vi "test_Adding Static Scalar Input Channels.vi"(8 "error in (no error)":errorcluster, 11 "TestCase in":refnum<class "FPGA Addon Adding a Channel Item.lvclass">) -> (0 "error out":errorcluster, 3 "TestCase out":refnum<class "FPGA Addon Adding a Channel Item.lvclass">)   [LabVIEW 2019, in "FPGA Addon Adding a Channel Item.lvclass"]
uses:
  FPGA Addon Adding a Channel Item.lvclass
  <vilib>/NI VeriStand/Custom Device API/Custom Device Channel.ctl
  <vilib>/NI VeriStand/Custom Device API/Custom Device Channel Type.ctl
  Addon/Addon Shared/Types/FG Action.ctl
  Addon/Addon System Explorer/Types/Channel Type.ctl
  FPGA Addon Adding a Channel Item.lvclass/FPGA Addon Adding a Channel Item.ctl
  Addon/Addon Shared/SubVIs/Constants.vi
  <vilib>/NI VeriStand/Custom Device Tools/Custom Device Utility Library/NI VeriStand - Search for Item by GUID.vi
  <vilib>/NI/NI VeriStand Advanced SysDef API/SysDef API/SysDef.Property.Get.vi
  <vilib>/NI/NI VeriStand Advanced SysDef API/_SubVIs/SysDef.Property.Get.Variant.vi
  <vilib>/NI/NI VeriStand Advanced SysDef API/SysDef API/SysDef.Property.Set.vi
  <vilib>/NI/NI VeriStand Advanced SysDef API/_SubVIs/SysDef.Property.Set.Variant.vi
  <vilib>/NI/NI VeriStand Advanced SysDef API/_SubVIs/SysDef.Search.GUIDs.vi
  <vilib>/addons/_JKI Toolkits/VI Tester/TestCase.llb/TestCase.lvclass
  Addon/Addon System Explorer/FPGA Addon System Explorer.lvlib
  Addon/Addon Shared/FPGA Addon Shared.lvlib
  <vilib>/NI VeriStand/Custom Device Tools/Custom Device Utility Library/Custom Device Utility Library.lvlib
  <vilib>/NI/NI VeriStand Advanced SysDef API/SysDef API/Advanced System Definition.lvlib
  <vilib>/NI VeriStand/Custom Device API/Custom Device API.lvlib
  C:/Program Files (x86)/National Instruments/LabVIEW 2019/vi.lib/addons/_JKI Toolkits/VI Tester/TestCase.llb/TestCase.lvclass
panel:
  out "GUIDs":string[](array[string])
  out "Channels":T1[](array[typedef])
  in  "remove":bool
  in  "add":bool
  out "Names":string[](array[string])
  in  "Available Registers":i32[](listbox)
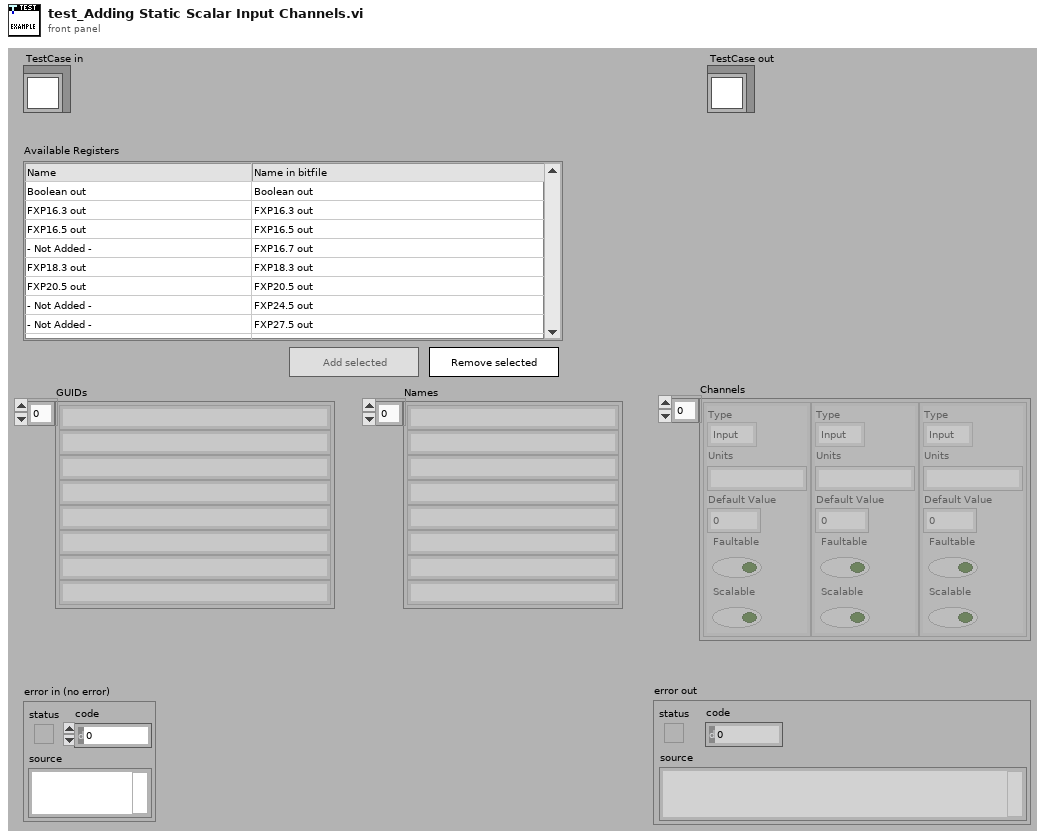
[diagram p1: front panel]
types:
  T1 = typedef "Custom Device API.lvlib/Custom Device Channel.ctl" = cluster{"Type":T2, "Units":string, "Default Value":dbl, "Faultable":bool, "Scalable":bool}
  T2 = typedef "Custom Device API.lvlib/Custom Device Channel Type.ctl" = enum16{"Input", "Output"}
  T3 = typedef "FPGA Addon System Explorer.lvlib/Channel Type.ctl" = enum16{"Write Channel", "Read Channel", "Write Waveform", "Read Waveform"}
  T4 = typedef "FPGA Addon Shared.lvlib/FG Action.ctl" = enum8{"GET", "SET"}
  T5 = typedef "Custom Device API.lvlib/Custom Device Item Ref.ctl" = u64
  T6 = typedef "FPGA Addon Shared.lvlib/Register Information.ctl" = cluster{"Name":string, "Data Type":T7, "Default Value":variant}
  T7 = typedef "FPGA Addon Shared.lvlib/Data Type.ctl" = enum8{"<Null>", "I8", "I16", "I32", "I64", "U8", "U16", "U32", "U64", "SGL", "Boolean", "Analog PWM In Settings", "Analog PWM In", "Digital PWM In Settings", "Digital PWM In", "Digital PWM Out", "Sine Out", "FXP+/-24.5", "FXP+/-16.5", "FXP+/-32.8", "FXP+/-64.32", "FXP+/-16.7", "FXP+/-20.5", "FXP+/-27.5", "FXP+/-32.16", "FXP+16.3", "FXP+18.3", "Digital Static In", "Digital Static Out", "Digital Static In Settings", "Digital WSS Out", "Quad Encoder Settings", "Quad Encoder In", "Group"}
  T8 = typedef "FPGA Addon System Explorer.lvlib/Listbox Cluster.ctl" = cluster{"add":refnum<vi>, "remove":refnum<vi>, "Listbox":refnum<vi>, "selected":i32[], "not present":i32[], "listbox text":string[][], "Section Ref":T5}
  T9 = typedef "Advanced System Definition.lvlib/TreeItem.Info.ctl" = cluster{"Name":string, "Description":string, "GUID":string, "Is Channel":bool, "Channel":T1, "Is Waveform":bool, "Waveform":T10}
  T10 = typedef "Custom Device API.lvlib/Custom Device Waveform.ctl" = cluster{"Data Type":T11, "Units":string}
  T11 = typedef "Custom Device API.lvlib/Custom Device Waveform DataType.ctl" = enum16{"Double", "Complex Double"}
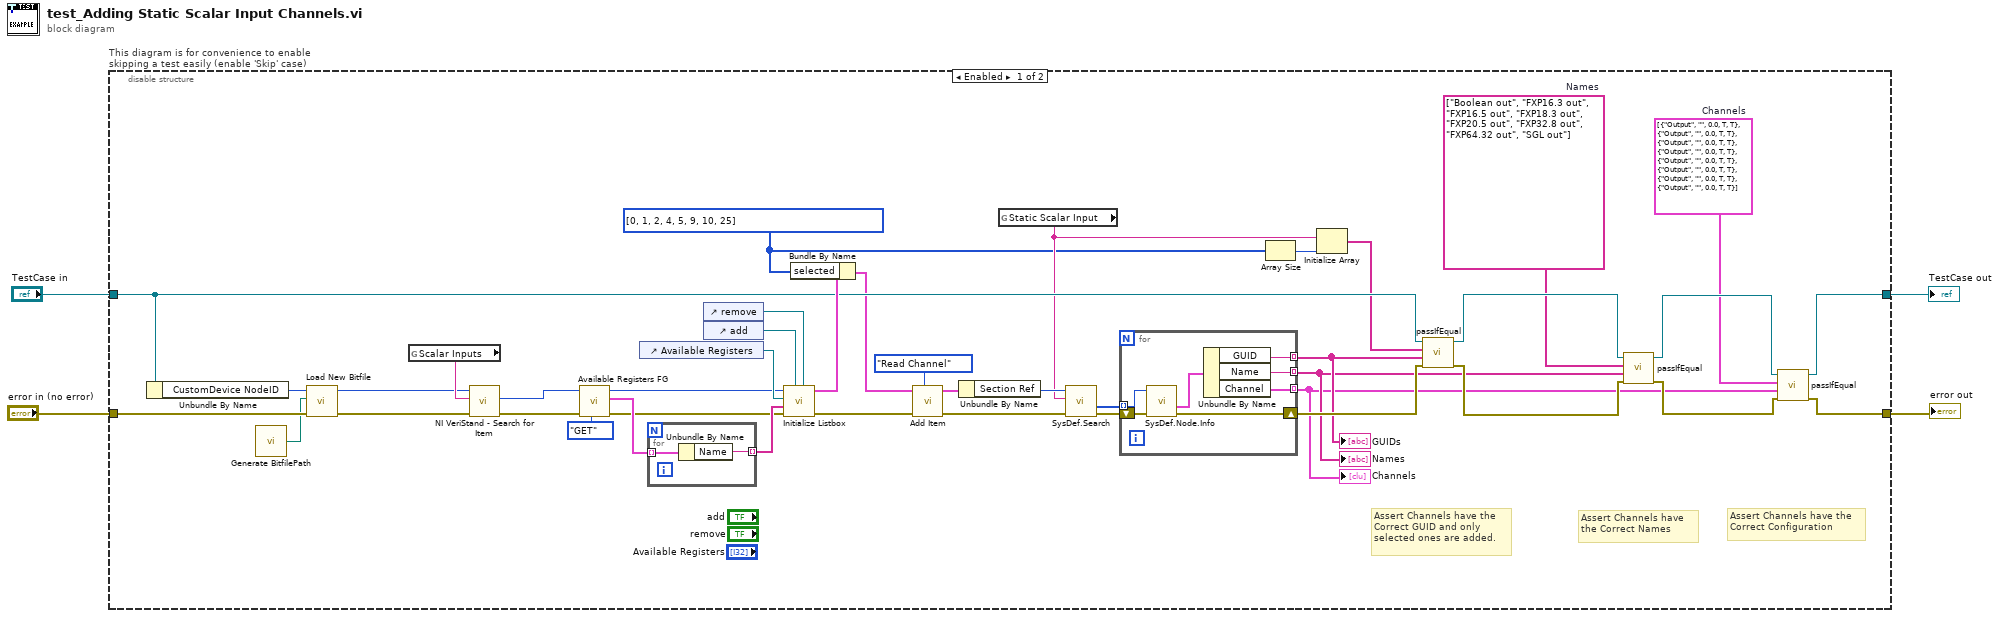
[diagram p0: block diagram]
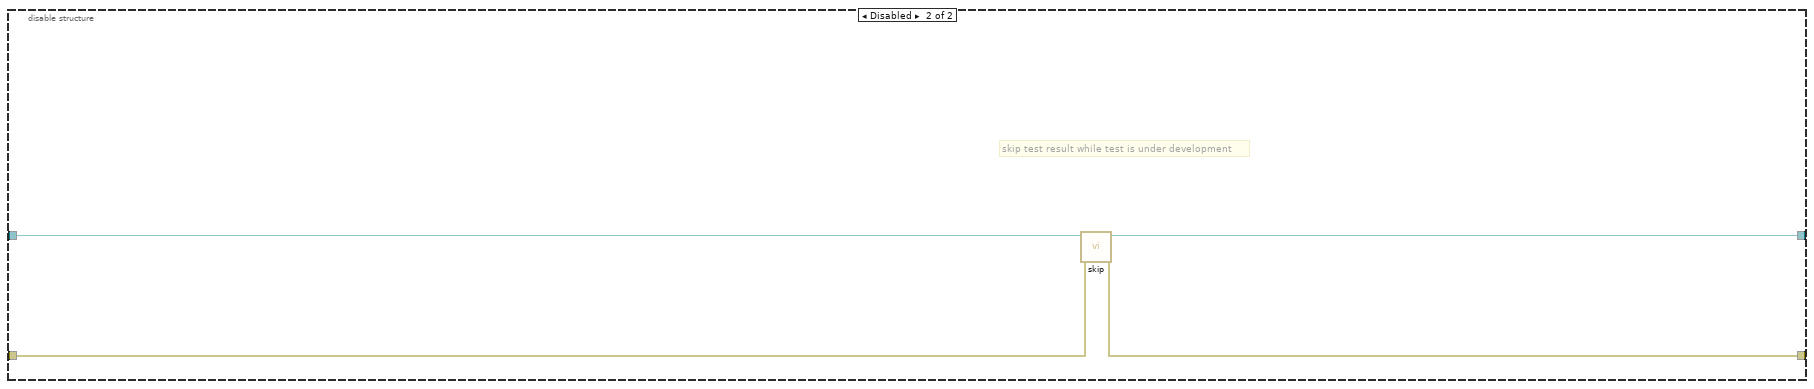
[diagram p2: hidden frame]
diagram:
  n1 = disable-structure "This diagram is for convenience to enable skipping a test easily (enable 'Skip' case)" shown="Enabled" {
    disable-tunnel: "TestCase in" -> [w26 w59]
    disable-tunnel: [w22 w57] -> w1
    disable-tunnel: [w19 w58] -> w3
    disable-tunnel: "error in (no error)" -> [w15 w56]
    frame Enabled {
      w17 = T1[] [{"Type"=enum."Output", "Units"="", "Default Value"=0.0, "Faultable"=TRUE, "Scalable"=TRUE}, {"Type"=enum."Output", "Units"="", "Default Value"=0.0, "Faultable"=TRUE, "Scalable"=TRUE}, {"Type"=enum."Output", "Units"="", "Default Value"=0.0, "Faultable"=TRUE, "Scalable"=TRUE}, {"Type"=enum."Output", "Units"="", "Default Value"=0.0, "Faultable"=TRUE, "Scalable"=TRUE}, {"Type"=enum."Output", "Units"="", "Default Value"=0.0, "Faultable"=TRUE, "Scalable"=TRUE}, {"Type"=enum."Output", "Units"="", "Default Value"=0.0, "Faultable"=TRUE, "Scalable"=TRUE}, {"Type"=enum."Output", "Units"="", "Default Value"=0.0, "Faultable"=TRUE, "Scalable"=TRUE}, {"Type"=enum."Output", "Units"="", "Default Value"=0.0, "Faultable"=TRUE, "Scalable"=TRUE}]  # Channels
      w23 = string[] ["Boolean out", "FXP16.3 out", "FXP16.5 out", "FXP18.3 out", "FXP20.5 out", "FXP32.8 out", "FXP64.32 out", "SGL out"]  # Names
      w6 = i32[] [0, 1, 2, 4, 5, 9, 10, 25] ("selected")
      # "Assert Channels have the Correct Configuration"
      # "Assert Channels have the Correct Names"
      # "Assert Channels have the Correct GUID and only selected ones are added."
      n2 = Unbundle By Name(w26) -> ("CustomDevice NodeID"=w14:u64)
      n3 = call "Generate BitfilePath.vi"() -> ("Bitfile path"=w13:path)
      n4 = call "Load New Bitfile.vi"("error in (no error)"=w15, "NewVal"=w13, "Item Ref in"=w14) -> ("error out"=w16:errorcluster, "Section Ref out"=w12:T5)  [unwired: 7 in]
      n5 = global read "Constants.vi" "Scalar Inputs"() -> (w40:string)
      n6 = call-poly <vilib>:"NI VeriStand - Search for Item.vi"("error in"=w16, "Item GUID"=w40, "Section Ref in"=w12) -> ("error out"=w39:errorcluster, "Item Ref"=w34:T5)  [unwired: 5 in, 2 out]
      n7 = call "Available Registers FG.vi"("Action"=FG_Action."GET", "error in (no error)"=w39, "Item Ref"=w34) -> ("error out"=w38:errorcluster, "Available Registers"=w44:T6[], "Item Ref out"=w36:T5)  [unwired: 6 in]
      n8 = control-ref of="Available Registers"() -> (w46:refnum<vi>)
      n9 = for {
        tunnel: w44 -> [w48] mode=indexing
        tunnel: [w47] -> w43 mode=indexing
        n10 = Unbundle By Name(w48) -> ("Name"=w47:string)
      }
      n11 = control-ref of="remove"() -> (w31:refnum<vi>)
      n12 = control-ref of="add"() -> (w32:refnum<vi>)
      n13 = call "Initialize Listbox.vi"("remove"=w31, "add"=w32, "error in (no error)"=w38, "Names"=w43, "Listbox"=w46, "Item Ref"=w36) -> ("error out"=w37:errorcluster, "Listbox Refs"=w41:T8)  [unwired: 4 in]
      n14 = Bundle By Name(cluster=w41, "selected"=w6) -> (w10:T8)
      n15 = call "Add Item.vi"("Action"=Channel_Type."Read Channel", "error in (no error)"=w37, "Listbox Refs in"=w10) -> ("error out"=w11:errorcluster, "Listbox Refs out"=w9:T8)  [unwired: 7 in]
      n16 = Unbundle By Name(w9) -> ("Section Ref"=w33:T5)
      n17 = global read "Constants.vi" "Static Scalar Input"() -> (w7:string)
      n18 = call-poly <vilib>:"SysDef.Search.vi"("error in (no error)"=w11, "GUID"=w7, "nodeID"=w33) -> ("error out"=w35:errorcluster, "Values Out"=w30:u64[])  [unwired: 5 in, 2 out]
      n19 = for {
        tunnel: w30 -> [w51] mode=indexing
        tunnel: [w49] -> w24 mode=indexing
        tunnel: [w52] -> w18 mode=indexing
        tunnel: [w50] -> w27 mode=indexing
        shift-right: [w54] -> w28
        shift-left: w35 -> [w55]
        n20 = call <vilib>:"SysDef.Node.Info.vi"("error in (no error)"=w55, "nodeID"=w51) -> ("error out"=w54:errorcluster, "Item Info"=w53:T9)  [unwired: 6 in, 2 out]
        n21 = Unbundle By Name(w53) -> ("GUID"=w50:string, "Name"=w49:string, "Channel"=w52:T1)
      }
      "Names" <- w24
      "Channels" <- w18
      "GUIDs" <- w27
      n22 = Array Size(array=w6) -> (size(s)=w5:i32)
      n23 = Initialize Array(w7, w5) -> (w8:string[])
      n24 = call-dynamic "passIfEqual.vi"("error in (no error)"=w28, "y"=w27, "x"=w8, "TestCase in"=w26) -> ("error out"=w29:errorcluster, "TestCase out"=w25:refnum<class "FPGA Addon Adding a Channel Item.lvclass">)  [unwired: 6 in]
      n25 = call-dynamic "passIfEqual.vi"("error in (no error)"=w29, "y"=w24, "x"=w23, "TestCase in"=w25) -> ("error out"=w20:errorcluster, "TestCase out"=w21:refnum<class "FPGA Addon Adding a Channel Item.lvclass">)  [unwired: 6 in]
      n26 = call-dynamic "passIfEqual.vi"("error in (no error)"=w20, "y"=w18, "x"=w17, "TestCase in"=w21) -> ("error out"=w19:errorcluster, "TestCase out"=w22:refnum<class "FPGA Addon Adding a Channel Item.lvclass">)  [unwired: 6 in]
    }
    frame Disabled {
      # "skip test result while test is under development"
      n27 = call <vilib>:"skip.vi"("error in (no error)"=w56, "TestCase in"=w59) -> ("error out"=w58:errorcluster, "TestCase out"=w57:refnum<class "FPGA Addon Adding a Channel Item.lvclass">)  [unwired: 8 in]
    }
  }
  "error out" <- w3
  "TestCase out" <- w1
